vi "Initialize Driver.vi"(8 "error in (no error)":errorcluster, 11 "Section Ref in":T21 format="%.0x") -> (0 "error out":errorcluster, 3 "Vars":T1 {"OutgoingRegisters.Refs"."Data Type" format="%.0x"; "IncomingDMA.Refs"."Refs"."Data Type" format="%.0x"; "IncomingDMA.Refs"."DMA Settings"."DMA Host Buffer" items=["1 Second"=1, "2 Seconds"=2, "5 Seconds"=5, "10 Seconds"=10]; "IncomingDMA.Refs"."DMA Settings"."dt" format="%#_p"; "IncomingDMA.Refs"."DMA Settings"."Update Rate" items=["1 Hz"=1, "2 Hz"=2, "5 Hz"=5, "10 Hz"=10]; "IncomingRegisters.Refs"."Data Type" format="%.0x"; "OutgoingDMA.Refs"."Refs"."Data Type" format="%.0x"; "Compiled"."IncomingRegisters.Settings"."Register"."Data Type" format="%.0x"; "Compiled"."IncomingRegisters.Refs"."Refs"."Data Reference" format="%.0x"; "Compiled"."OutgoingRegisters.Settings"."Register"."Data Type" format="%.0x"; "Compiled"."OutgoingRegisters.Refs"."Refs"."Data Reference" format="%.0x"; "Compiled"."IncomingDMA.Settings"."Data Type" format="%.0x"; "Compiled"."IncomingDMA.Settings"."DMA.Settings"."DMA Host Buffer" items=["1 Second"=1, "2 Seconds"=2, "5 Seconds"=5, "10 Seconds"=10]; "Compiled"."IncomingDMA.Settings"."DMA.Settings"."dt" format="%#_p"; "Compiled"."IncomingDMA.Settings"."DMA.Settings"."Update Rate" items=["1 Hz"=1, "2 Hz"=2, "5 Hz"=5, "10 Hz"=10]; "Compiled"."OutgoingDMA.Settings"."Data Type" format="%.0x"; "Compiled"."OutgoingDMA.Settings"."DMA.Settings"."DMA Host Buffer" items=["1 Second"=1, "2 Seconds"=2, "5 Seconds"=5, "10 Seconds"=10]; "Compiled"."OutgoingDMA.Settings"."DMA.Settings"."dt" format="%#_p"; "Compiled"."OutgoingDMA.Settings"."DMA.Settings"."Update Rate" items=["1 Hz"=1, "2 Hz"=2, "5 Hz"=5, "10 Hz"=10]})   [LabVIEW 2015, in "FPGA Addon Engine.lvlib"]
uses:
  FPGA Addon Engine.lvlib
  <vilib>/NI Veristand/Custom Device API/Custom Device Item Ref.ctl
  Types/State Variables.ctl
  Types/Register Settings.ctl
  Shared/Data Type.ctl
  Shared/Scalar Type.ctl
  Types/DMA Input References.ctl
  <vilib>/NI Veristand/Custom Device Waveform API/Multiple Waveforms Write (DBL)/Multiple Waveforms Write (DBL).lvclass
  Shared/DMA Settings.ctl
  Shared/Delacing Scheme.ctl
  Shared/DMA Acquisition Mode.ctl
  Types/DMA Input Refs.ctl
  Types/DMA Output References.ctl
  <vilib>/NI Veristand/Custom Device Waveform API/Single Waveform Read (DBL)/Single Waveform Read (DBL).lvclass
  Types/DMA Output Refs.ctl
  Shared/Compiled.Settings.ctl
  Shared/Compiled.RegisterSettings.ctl
  Shared/Register Information.ctl
  <vilib>/NI Veristand/Custom Device API/Block Data Reference.ctl
  <vilib>/NI Veristand/Custom Device API/Data Reference.ctl
  Shared/Compiled.DMASettings.ctl
  <vilib>/NI Veristand/Custom Device API/Waveform Data Reference.ctl
  Shared/FPGA Settings.ctl
  <vilib>/NI Veristand/Custom Device API/Custom Device Target Type.ctl
  Shared/FG Action.ctl
  Initialize Scalar Datatype Classes.vi
  <vilib>/NI Veristand/Custom Device API/NI VeriStand - Set Item Property.vi
  <vilib>/NI Veristand/Custom Device API/Set Item Property (String).vi
  <vilib>/NI Veristand/Custom Device API/Set Item Property (Path).vi
  <vilib>/NI Veristand/Custom Device API/Get Item Property (String).vi
  <vilib>/NI Veristand/Custom Device API/Get Item Property (Path).vi
  Shared/Constants.vi
  <vilib>/NI Veristand/Custom Device API/Get Item Property (Dependent File).vi
  <vilib>/NI Veristand/Custom Device API/Get Item Property (Variant).vi
  Shared/FPGA Addon Shared.lvlib
  <vilib>/NI VeriStand/Custom Device API/Custom Device API.lvlib
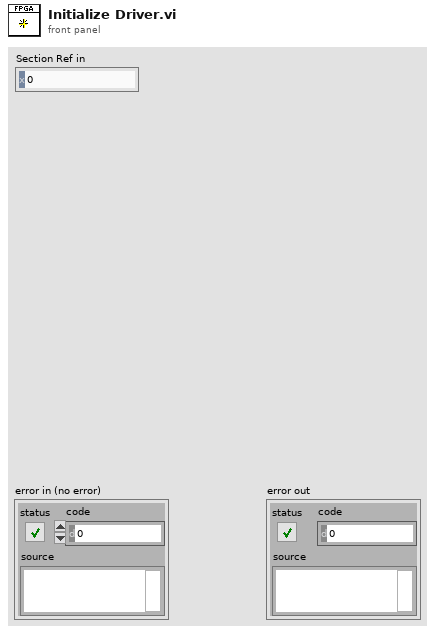
[diagram p1: front panel]
types:
  T1 = typedef "FPGA Addon Engine.lvlib/State Variables.ctl" = cluster{"FPGA Ref":refnum<k20>, "IncomingRegisters.Refs":T2[], "IncomingDMA.Refs":T5[], "OutgoingRegisters.Refs":T2[], "OutgoingDMA.Refs":T10[], "Compiled":T12}
  T2 = typedef "FPGA Addon Engine.lvlib/Register Settings.ctl" = cluster{"Data Type":T3, "U64":refnum<k20>, "U32":refnum<k20>, "U16":refnum<k20>, "U8":refnum<k20>, "I64":refnum<k20>, "I32":refnum<k20>, "I16":refnum<k20>, "I8":refnum<k20>, "SGL":refnum<k20>, "Bool":refnum<k20>, "Scalar Type":T4, "Index":i32, "Length":i32, "Analog PWM In":refnum<k20>, "Digital PWM In":refnum<k20>, "Digital PWM Out":refnum<k20>, "Analog PWM In Settings":refnum<k20>, "Digital PWM In Settings":refnum<k20>, "Sine Out":refnum<k20>, "FXP+/-24.5":refnum<k20>, "FXP+/-16.5":refnum<k20>, "FXP+/-32.8":refnum<k20>, "FXP+/-64.32":refnum<k20>, "FXP+/-16.7":refnum<k20>, "FXP+/-20.5":refnum<k20>, "FXP+/-27.5":refnum<k20>, "FXP+/-32.16":refnum<k20>, "Digital Static In":refnum<k20>, "Digital Static Out":refnum<k20>, "Digital Static In Settings":refnum<k20>, "Digital WSS Out":refnum<k20>}
  T3 = typedef "FPGA Addon Shared.lvlib/Data Type.ctl" = enum8{"<Null>", "I8", "I16", "I32", "I64", "U8", "U16", "U32", "U64", "SGL", "Boolean", "Analog PWM In Settings", "Analog PWM In", "Digital PWM In Settings", "Digital PWM In", "Digital PWM Out", "Sine Out", "FXP+/-24.5", "FXP+/-16.5", "FXP+/-32.8", "FXP+/-64.32", "FXP+/-16.7", "FXP+/-20.5", "FXP+/-27.5", "FXP+/-32.16", "Digital Static In", "Digital Static Out", "Digital Static In Settings", "Digital WSS Out"}
  T4 = typedef "FPGA Addon Shared.lvlib/Scalar Type.ctl" = enum16{"Standard", "Bitpacked"}
  T5 = typedef "FPGA Addon Engine.lvlib/DMA Input References.ctl" = cluster{"Waveform Ref":refnum<class "Multiple Waveforms Write (DBL).lvclass">, "Name":string, "DMA Settings":T6, "Refs":T9}
  T6 = typedef "FPGA Addon Shared.lvlib/DMA Settings.ctl" = cluster{"Number of Channels":u8, "Delacing Scheme":T7, "Update Rate":u32, "dt":dbl, "Mode":T8, "Number of Samples":u32, "DMA Host Buffer":u32}
  T7 = typedef "FPGA Addon Shared.lvlib/Delacing Scheme.ctl" = enum8{"Interleaved", "Bitpacked"}
  T8 = typedef "FPGA Addon Shared.lvlib/DMA Acquisition Mode.ctl" = enum8{"Continuous", "Triggered Finite"}
  T9 = typedef "FPGA Addon Engine.lvlib/DMA Input Refs.ctl" = cluster{"Data Type":T3, "DMA_SGL":refnum<k20>, "DMA_U64":refnum<k20>, "DMA_I64":refnum<k20>, "DMA_FXP+/-32.8":refnum<k20>, "DMA_FXP+/-64.32":refnum<k20>, "DMA_U32":refnum<k20>, "DMA_U16":refnum<k20>, "DMA_U8":refnum<k20>, "DMA_I32":refnum<k20>, "DMA_I16":refnum<k20>, "DMA_I8":refnum<k20>, "DMA_FXP+/-32.16":refnum<k20>}
  T10 = typedef "FPGA Addon Engine.lvlib/DMA Output References.ctl" = cluster{"Waveforms":refnum<class "Single Waveform Read (DBL).lvclass">[], "Name":string, "Refs":T11}
  T11 = typedef "FPGA Addon Engine.lvlib/DMA Output Refs.ctl" = cluster{"Data Type":T3, "DMA_SGL":refnum<k20>, "DMA_U64":refnum<k20>, "DMA_I64":refnum<k20>, "DMA_FXP+/-32.8":refnum<k20>, "DMA_FXP+/-64.32":refnum<k20>, "DMA_U32":refnum<k20>, "DMA_U16":refnum<k20>, "DMA_U8":refnum<k20>, "DMA_I32":refnum<k20>, "DMA_I16":refnum<k20>, "DMA_I8":refnum<k20>, "DMA_FXP+/-32.16":refnum<k20>}
  T12 = typedef "FPGA Addon Shared.lvlib/Compiled.Settings.ctl" = cluster{"Name":string, "IncomingRegisters.Settings":T13[], "IncomingRegisters.Refs":cluster{"Refs":T15[], "Values":dbl[]}, "OutgoingRegisters.Settings":T13[], "OutgoingRegisters.Refs":cluster{"Refs":T15[], "Values":dbl[]}, "Incoming.Size":i32, "Outgoing.Size":i32, "IncomingDMA.Settings":T17[], "OutgoingDMA.Settings":T17[], "FPGA.Settings":T19, "Target.Type":T20}
  T13 = typedef "FPGA Addon Shared.lvlib/Compiled.RegisterSettings.ctl" = cluster{"Scalar Type":T4, "Index":i32, "Length":i32, "Register":T14}
  T14 = typedef "FPGA Addon Shared.lvlib/Register Information.ctl" = cluster{"Name":string, "Data Type":T3, "Default Value":variant}
  T15 = typedef "Custom Device API.lvlib/Block Data Reference.ctl" = cluster{"Data Reference":T16, "Offset":u64, "Length":u64}
  T16 = typedef "Custom Device API.lvlib/Data Reference.ctl" = i32
  T17 = typedef "FPGA Addon Shared.lvlib/Compiled.DMASettings.ctl" = cluster{"Name":string, "Data Type":T3, "DMA.Settings":T6, "DMA.VSRefs":T18[]}
  T18 = typedef "Custom Device API.lvlib/Waveform Data Reference.ctl" = i32
  T19 = typedef "FPGA Addon Shared.lvlib/FPGA Settings.ctl" = cluster{"Bitfile path":path, "RIO Device Address":string}
  T20 = typedef "Custom Device API.lvlib/Custom Device Target Type.ctl" = enum16{"PharLap", "VxWorks", "Windows", "Linux_32_ARM", "Linux_x64"}
  T21 = typedef "Custom Device API.lvlib/Custom Device Item Ref.ctl" = u64
  T22 = typedef "FPGA Addon Shared.lvlib/FG Action.ctl" = enum8{"GET", "SET"}
  T23 = typedef "Custom Device API.lvlib/Dependent File Optional Info.ctl" = cluster{"Version":string, "RTDestination":path, "ForceDownload":bool, "SupportedTarget":string, "MD5":string}
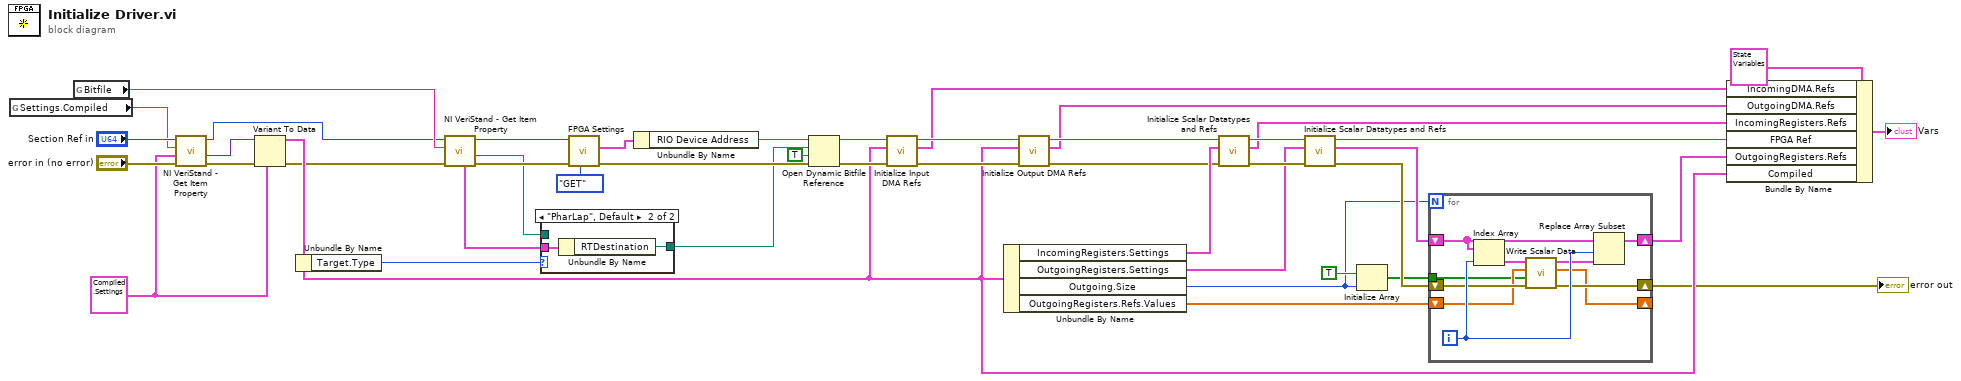
[diagram p0: block diagram]
diagram:
  w13 = T12 {"Name"="", "IncomingRegisters.Settings"=[], "IncomingRegisters.Refs"={"Refs"=[], "Values"=[]}, "OutgoingRegisters.Settings"=[], "OutgoingRegisters.Refs"={"Refs"=[], "Values"=[]}, "Incoming.Size"=0, "Outgoing.Size"=0, "IncomingDMA.Settings"=[], "OutgoingDMA.Settings"=[], "FPGA.Settings"={"Bitfile path"=path "", "RIO Device Address"=""}, "Target.Type"=enum."PharLap"} ("Settings.Compiled")
  n1 = global read "Constants.vi" "Settings.Compiled"() -> (w15:string)
  n2 = global read "Constants.vi" "Bitfile"() -> (w38:string)
  n3 = call-poly <vilib>:"NI VeriStand - Get Item Property.vi"("error in (no error)"="error in (no error)", "Default Value"=w13, "Property Name"=w15, "Item Ref in"="Section Ref in") -> ("error out"=w16:errorcluster, "Value"=w14:variant, "Item Ref out"=w9:T21)  [unwired: 4 in, 1 out]
  n4 = Variant To Data(error in=w16, type=w13, Variant=w14) -> (data=w12:T12, error out=w10:errorcluster)
  n5 = Unbundle By Name(w12) -> ("Target.Type"=w11:T20)
  n6 = call-poly <vilib>:"NI VeriStand - Get Item Property.vi"("error in (no error)"=w10, "Property Name"=w38, "Item Ref in"=w9) -> ("error out"=w36:errorcluster, "Path"=w33:path, "Item Ref out"=w37:T21, "OptionalInfo"=w35:T23)  [unwired: 4 in, 1 out]
  n7 = case shown="\"PharLap\", Default" w11 {
    tunnel: w35 -> [_ w48]
    tunnel: [w46 w47] -> w34
    tunnel: w33 -> [w46 _]
    frame "Windows" {
    }
    frame "PharLap", Default {
      n8 = Unbundle By Name(w48) -> ("RTDestination"=w47:path)
    }
  }
  n9 = call "FPGA Settings.vi"("Action"=FG_Action."GET", "error in (no error)"=w36, "Item Ref"=w37) -> ("error out"=w44:errorcluster, "FPGA Settings"=w42:T19)  [unwired: 6 in, 1 out]
  n10 = Unbundle By Name(w42) -> ("RIO Device Address"=w41:string)
  n11 = Open Dynamic Bitfile Reference(0:w41, 1:w34, 2:TRUE ("Run When Loaded"), 3:w44) -> (5:w31:refnum<k20>, 8:w32:errorcluster)  [unwired: 1 in]
  n12 = call "Initialize Input DMA Refs.vi"("error in (no error)"=w32, "Settings.Compiled"=w12, "FPGA Ref"=w31) -> ("error out"=w23:errorcluster, "DMA Settings"=w21:T5[], "FPGA Ref"=w26:refnum<k20>)  [unwired: 6 in]
  n13 = Unbundle By Name(w12) -> ("IncomingRegisters.Settings"=w28:T13[], "OutgoingRegisters.Settings"=w27:T13[], "Outgoing.Size"=w1:i32, "OutgoingRegisters.Refs.Values"=w5:dbl[])
  n14 = call "Initialize Output DMA Refs.vi"("error in (no error)"=w23, "Settings.Compiled"=w12, "FPGA Ref"=w26) -> ("error out"=w24:errorcluster, "DMA"=w20:T10[], "FPGA Ref"=w25:refnum<k20>)  [unwired: 6 in]
  n15 = call "Initialize Scalar Datatypes and Refs.vi"("error in (no error)"=w24, "Registers"=w28, "FPGA Ref"=w25) -> ("error out"=w30:errorcluster, "Registers Ref"=w19:T2[], "FPGA Ref"=w29:refnum<k20>)  [unwired: 6 in]
  n16 = call "Initialize Scalar Datatypes and Refs.vi"("error in (no error)"=w30, "Registers"=w27, "FPGA Ref"=w29) -> ("error out"=w7:errorcluster, "Registers Ref"=w8:T2[], "FPGA Ref"=w22:refnum<k20>)  [unwired: 6 in]
  n17 = Initialize Array(TRUE, w1) -> (w3:bool[])
  n18 = for {
    N: w1 -> [_]
    shift-right: [w50] -> _
    shift-left: w5 -> [w51]
    shift-right: [w58] -> w2
    shift-left: w8 -> [w57]
    shift-right: [w53] -> w6
    shift-left: w7 -> [w54]
    tunnel: w3 -> [w49]
    i -> [w56]
    n19 = Index Array(array=w57, index=w56) -> (element=w52:T2)
    n20 = call "Write Scalar Data.vi"("error in (no error)"=w54, "Changed?"=w49, "Values"=w51, "Cluster"=w52) -> ("error out"=w53:errorcluster, "Values"=w50:dbl[], "Cluster"=w55:T2)  [unwired: 5 in]
    n21 = Replace Array Subset(array=w57, new element=w55, index=w56) -> (w58:T2[])
  }
  "error out" <- w6
  n22 = Bundle By Name(cluster=T1 {"FPGA Ref"=refnum, "IncomingRegisters.Refs"=[], "IncomingDMA.Refs"=[], "OutgoingRegisters.Refs"=[], "OutgoingDMA.Refs"=[], "Compiled"={"Name"="", "IncomingRegisters.Settings"=[], "IncomingRegisters.Refs"={"Refs"=[], "Values"=[]}, "OutgoingRegisters.Settings"=[], "OutgoingRegisters.Refs"={"Refs"=[], "Values"=[]}, "Incoming.Size"=0, "Outgoing.Size"=0, "IncomingDMA.Settings"=[], "OutgoingDMA.Settings"=[], "FPGA.Settings"={"Bitfile path"=path "", "RIO Device Address"=""}, "Target.Type"=enum."PharLap"}}, "IncomingDMA.Refs"=w21, "OutgoingDMA.Refs"=w20, "IncomingRegisters.Refs"=w19, "FPGA Ref"=w22, "OutgoingRegisters.Refs"=w2, "Compiled"=w12) -> (→"Vars":T1)
